vi "N5700 Close.vi"(5 "error":errorcluster, 8 "VISA name":refnum<visa-resource-name>) -> (0 "error out":errorcluster)   [LabVIEW 2020]
doc: "This VI closes the I/O interface with the Agilent N5700 Power Supply."
panel:
  # "Agilent Technologies  \nSeries N5700A\n  DC Power Supplies"
  # "Close Instrument Port"
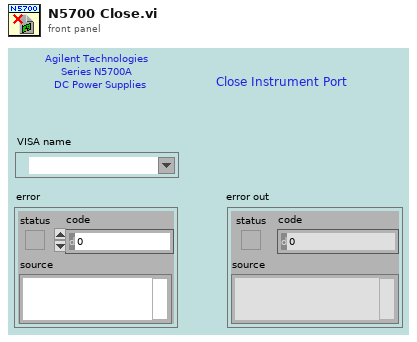
[diagram p1: front panel]
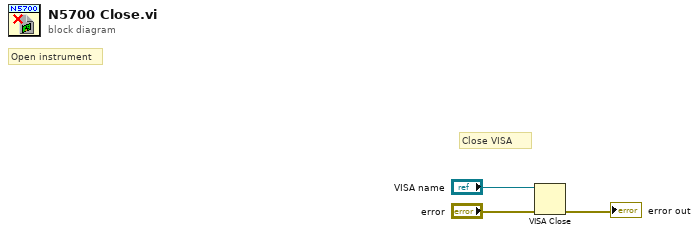
[diagram p0: block diagram]
diagram:
  # "Close VISA"
  # "Open instrument"
  n1 = VISA Close(VISA resource name="VISA name", error in (no error)="error") -> (error out=→"error out":errorcluster)
